vi "Log Data to File.vi"(8 "Error In":errorcluster, 11 "Log File Path":path) -> (0 "Error Out":errorcluster)   [LabVIEW 2019]
uses:
  <vilib>/express/express signal manip/GetorSetDDTAttributes/Shared VIs/TimeType.ctl
  WSData.vi
  <vilib>/express/express signal manip/GetorSetDDTAttributes/Shared VIs/TimeMode Enum to Boolean.vi
  <vilib>/express/express shared/transition.llb/Dynamic To Waveform Array.vi
  <vilib>/express/express signal manip/GetorSetDDTAttributes/Set DDT Attributes/SetT0.vi
  <vilib>/express/express signal manip/GetorSetDDTAttributes/Set DDT Attributes/sub Set StartTimeStamp.vi
  <vilib>/express/express shared/transition.llb/Waveform Array To Dynamic.vi
  <vilib>/express/express signal manip/GetorSetDDTAttributes/Set DDT Attributes/Set DDT Properties.xnode
  <vilib>/express/express signal manip/GetorSetDDTAttributes/Shared VIs/GetSetShared.lvlib
  <vilib>/express/express signal manip/GetorSetDDTAttributes/Set DDT Attributes/Set DDT Attributes.lvlib
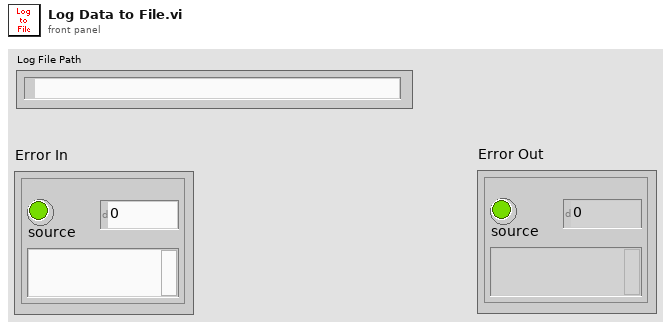
[diagram p1: front panel]
types:
  T1 = cluster{"TagId":string, "TagName":string, "TagType":string, "PhysicalChannel":tag, "Vmin":dbl, "Vmax":dbl, "Unit":string, "EUmin":dbl, "EUmax":dbl}[]
  T2 = typedef "GetSetShared.lvlib/TimeType.ctl" = enum16{"Absolute", "Relative"}
  T3 = typedef "Logging Settings.ctl" = cluster{"Logging Interval [s]":dbl, "Use Lowpass Filter":bool, "Tf [s]":dbl, "Logging Data to File":bool, "Log Folder":path, "Logging Data to Cloud Service":bool, "Data Cloud Service Url":string, "Use Random Data":bool}
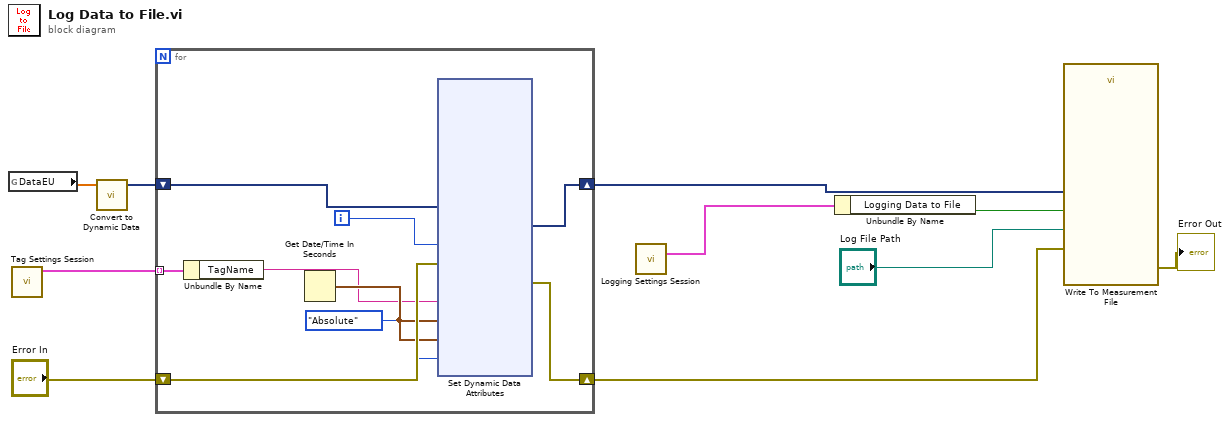
[diagram p0: block diagram]
diagram:
  n1 = global read "WSData.vi" "DataEU"() -> (w2:dbl[])
  n2 = call "Tag Settings Session.vi"() -> ("Tag Settings"=w7:T1)  [unwired: 10 in, 1 out]
  n3 = call "Convert to Dynamic Data"("Array"=w2) -> ("Dynamic Data Type"=w6:dynamicdata)  [unwired: 3 in]
  n4 = for {
    shift-right: [w11] -> w5
    shift-left: w6 -> [w12]
    tunnel: w7 -> [w14] mode=indexing
    shift-right: [w18] -> w9
    shift-left: "Error In" -> [w19]
    i -> [w17]
    n5 = Unbundle By Name(w14) -> ("TagName"=w13:string)
    n6 = Get Date/Time In Seconds() -> (seconds since 1Jan1904=w16:timestamp)
    n7 = xnode "Set Dynamic Data Attributes"("Signals In"=w12, "Signal Index"=w17, "error in"=w19, "Signal Name"=w13, "Start Timestamp"=w16, "Timestamp"=w16, "Time Mode"=TimeType."Absolute") -> ("Signals Out"=w11:dynamicdata, "error out"=w18:errorcluster)
  }
  n8 = call "Logging Settings Session.vi"() -> ("Logging Settings"=w4:T3)  [unwired: 14 in, 1 out]
  n9 = Unbundle By Name(w4) -> ("Logging Data to File"=w3:bool)
  n10 = call "Write To Measurement File"("Signals"=w5, "Enable"=w3, "error in (no error)"=w9, "Filename"="Log File Path") -> ("error out"=→"Error Out":errorcluster)  [unwired: 13 in, 2 out]
